vi "P3.2.vi"() -> ()   [LabVIEW 2020]
uses:
  <vilib>/Analysis/2dsp.llb/Real FFT.vi
  <vilib>/Analysis/2dsp.llb/Inverse Real FFT.vi
  <vilib>/Analysis/NI_AALPro.lvlib
panel:
  out "X 2":dbl[](array[numeric])
  out "X":dbl[](array[numeric])
  out "FFT {X}":cdb[](array[numeric])
  in  "FFT size":i32=-1
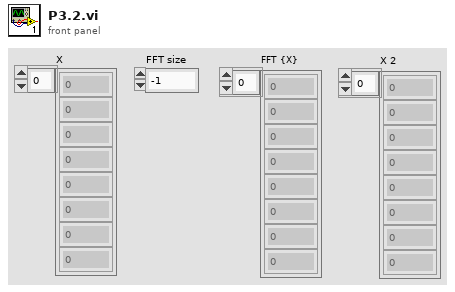
[diagram p1: front panel]
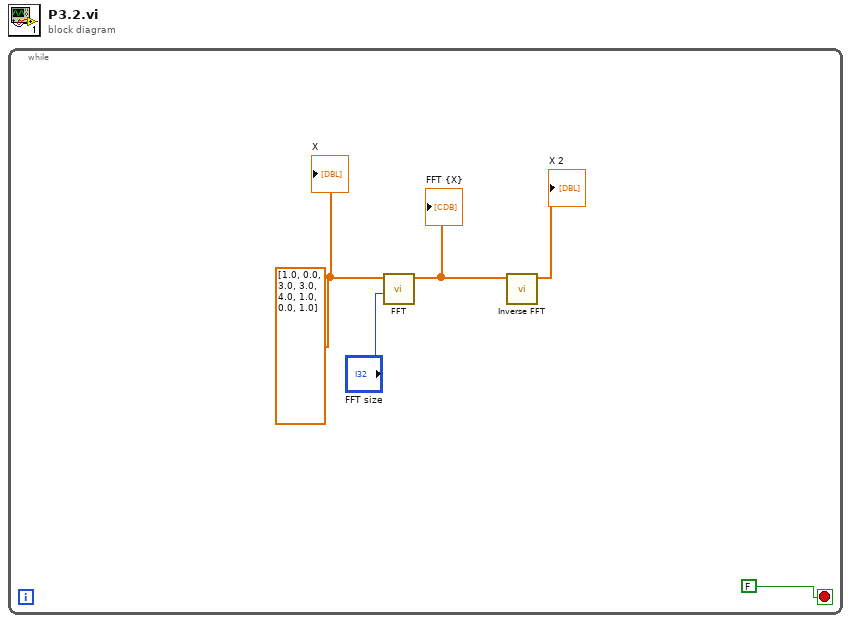
[diagram p0: block diagram]
diagram:
  n1 = while {
    stop <- FALSE ("stop") stop-if-true
    w5 = dbl[] [1.0, 0.0, 3.0, 3.0, 4.0, 1.0, 0.0, 1.0] ("X")
    n2 = call-poly <vilib>:"FFT.vi"("FFT size"="FFT size", "X"=w5) -> ("FFT {X}"=w2:cdb[])  [unwired: 8 in, 1 out]
    "FFT {X}" <- w2
    n3 = call-poly <vilib>:"Inverse FFT.vi"("FFT {X}"=w2) -> ("X"=→"X 2":dbl[])  [unwired: 9 in, 1 out]
    "X" <- w5
  }
